vi "AllianceDriverStationGet.vi"() -> (3 "Position":i32)   [LabVIEW 2023]
uses:
  AllianceColorGlobal.vi
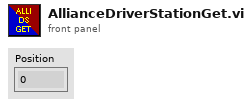
[diagram p1: front panel]
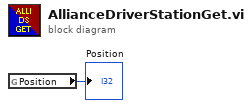
[diagram p0: block diagram]
diagram:
  n1 = global read "AllianceColorGlobal.vi" "Position"() -> (→"Position":i32)
